vi "Lockin_Amplifier_save_diag.vi"(0 "Reference signal (dialog if empty)":path=path "D:/#Meresek/Malaria/Malaria_measurement_program/Labview/Lock_in_Amplifier/tesztsor/timetrace_46.txt", 1 "averaging time":dbl=1.0 format="%0.2p", 2 "tolerance (Deviation)":dbl=3.0, 5 "Sample Number":i32=100000, 7 "dt":dbl=0.0002, 9 "Window (s)":dbl=3.0, 11 "Resolution":dbl=1e-05, 12 "Error In":errorcluster) -> (3 "LD_RMS":dbl, 4 "Lock-in R":cluster{dbl[], "Result":dbl[]}(graph), 6 "Lock-in Theta":cluster{dbl[], "Result":dbl[]}(graph), 8 "LD mean (V)":dbl format="%0.6f", 10 "LD deviation (V)":dbl format="%0.6f", 13 "dLD_RMS":dbl, 14 "Error Out":errorcluster, 15 "Integral":cluster{dbl[], dbl[]}[](graph))   [LabVIEW 2011]
uses:
  <vilib>/Utility/file.llb/Read From Spreadsheet File (DBL).vi
  <vilib>/Utility/file.llb/Write To Spreadsheet File (DBL).vi
  <vilib>/gmath/NI_Gmath.lvlib
  <vilib>/Analysis/NI_AALBase.lvlib
panel:
  in  "Tab Control":T1(tab)
  out "Reference signal / PLL Signal":cluster{"all rows":dbl[], "all rows":dbl[]}[](graph)
  out "Reference Spectrum":cluster{"f0":dbl, "df":dbl, "magnitude":dbl[]}(graph)
  out "Synthetized Spectrum":cluster{"f0":dbl, "df":dbl, "magnitude":dbl[]}(graph)
  in  "t0_ref":dbl
  in  "t0_LD":dbl=0.0001
  in  "Sampling Freq":dbl=5000.0
  in  "Cutoff Frequency":dbl=500.0
  out "Averaging window":dbl
  in  "SAVE":path=path "D:/#Meresek/Malaria/Malaria_measurement_program/Labview/Lock_in_Amplifier/tesztsor/timetrace_46.txt"
  out "LD Spectrum":cluster{"f0":dbl, "df":dbl, "magnitude":dbl[]}(graph)
  out "LD Signal":cluster{"all rows":dbl[], "all rows":dbl[]}[](graph)
  out "Signal Spectrum":cluster{"f0":dbl, "df":dbl, "magnitude":dbl[]}[](graph)
  out "Time Domain Signal":cluster{"xi used":dbl[], "yi":dbl[]}[](graph)
  out "Tolerance Level":dbl
  out "average":dbl
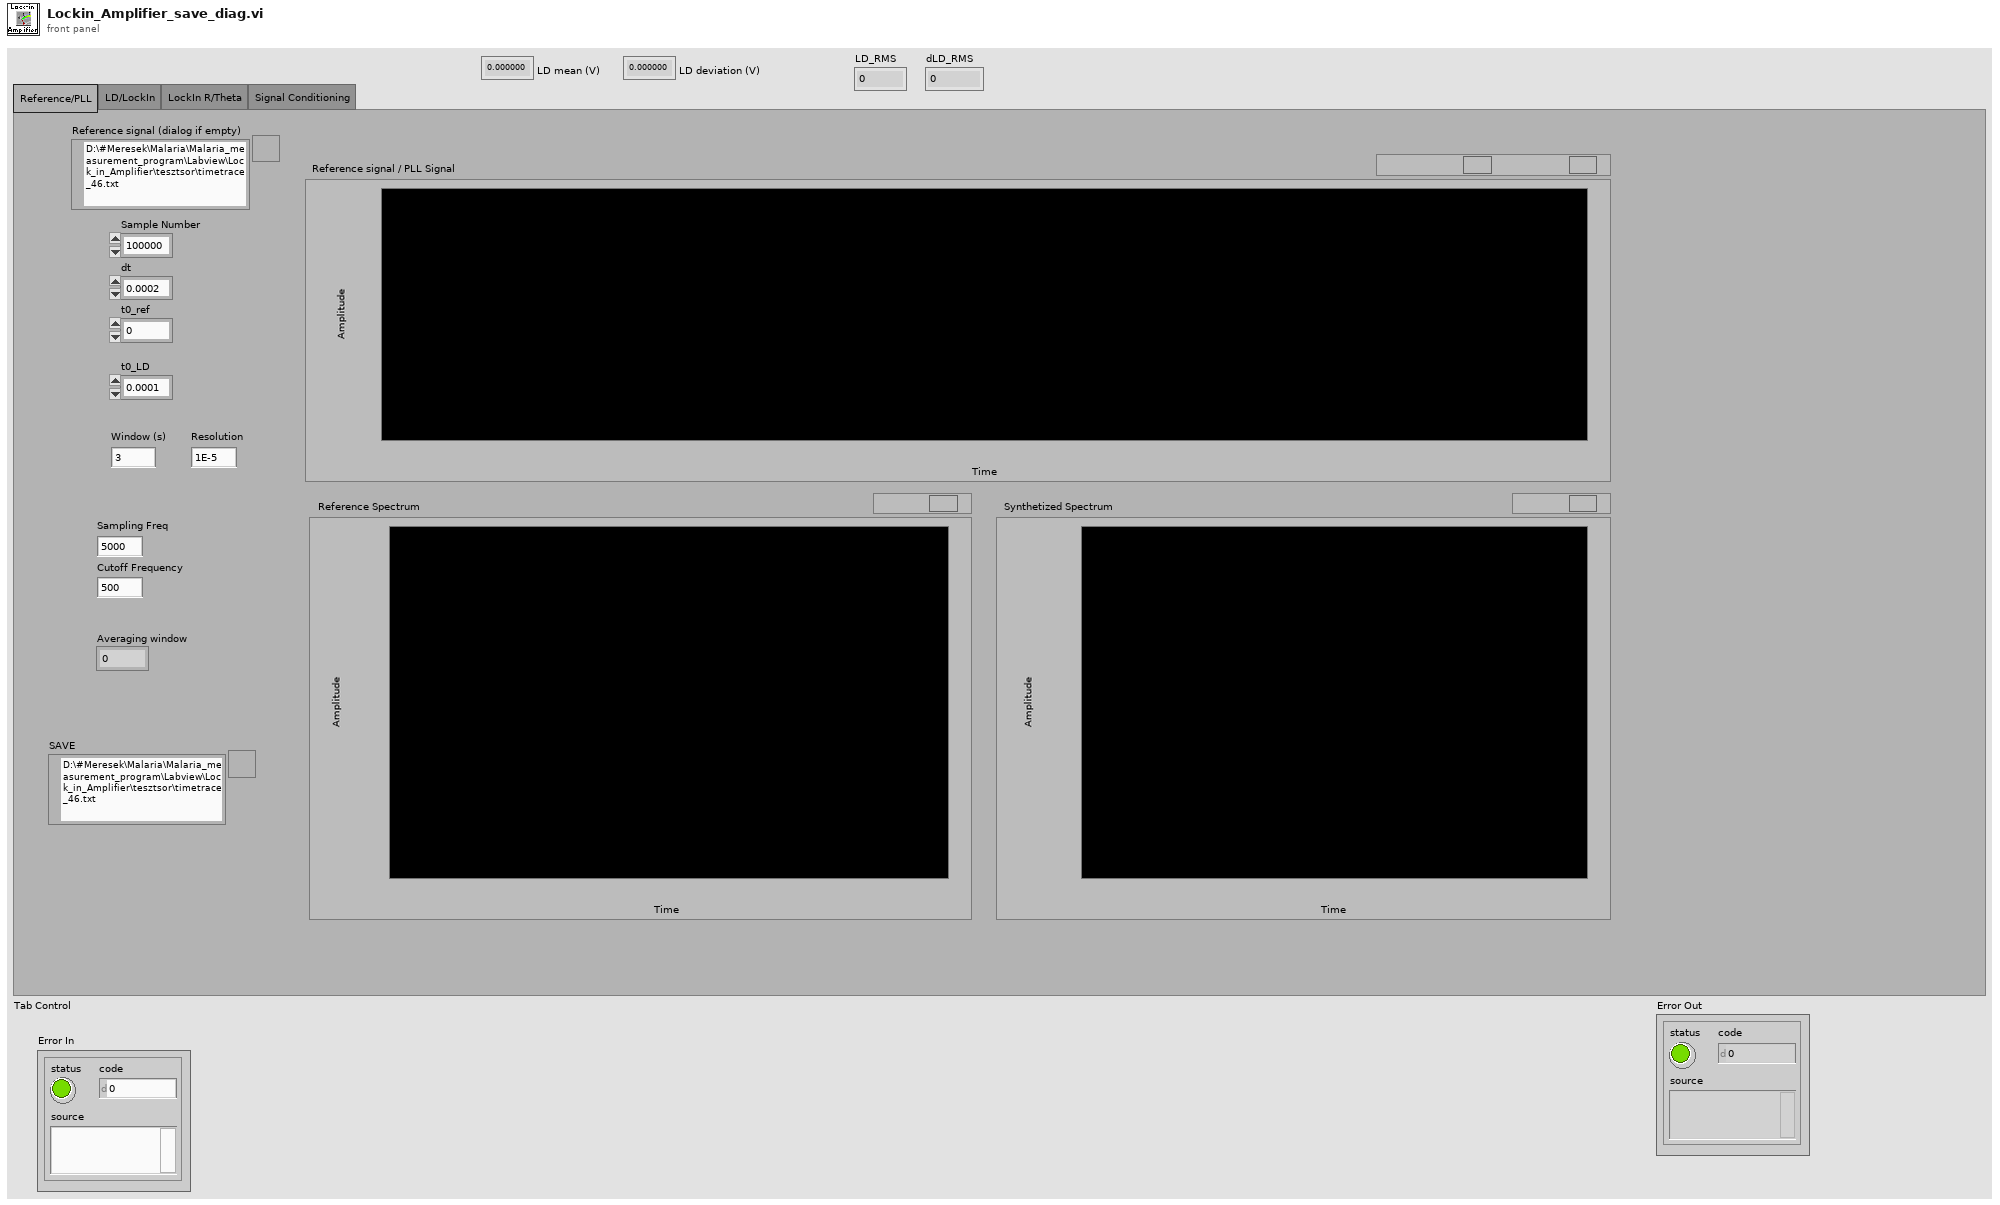
[diagram p1: front panel]
types:
  T1 = enum32{"Reference/PLL", "LD/LockIn", "LockIn R/Theta", "Signal Conditioning"}
  T2 = enum16{"open", "replace", "create", "open or create", "replace or create", "replace or create with confirmation"}
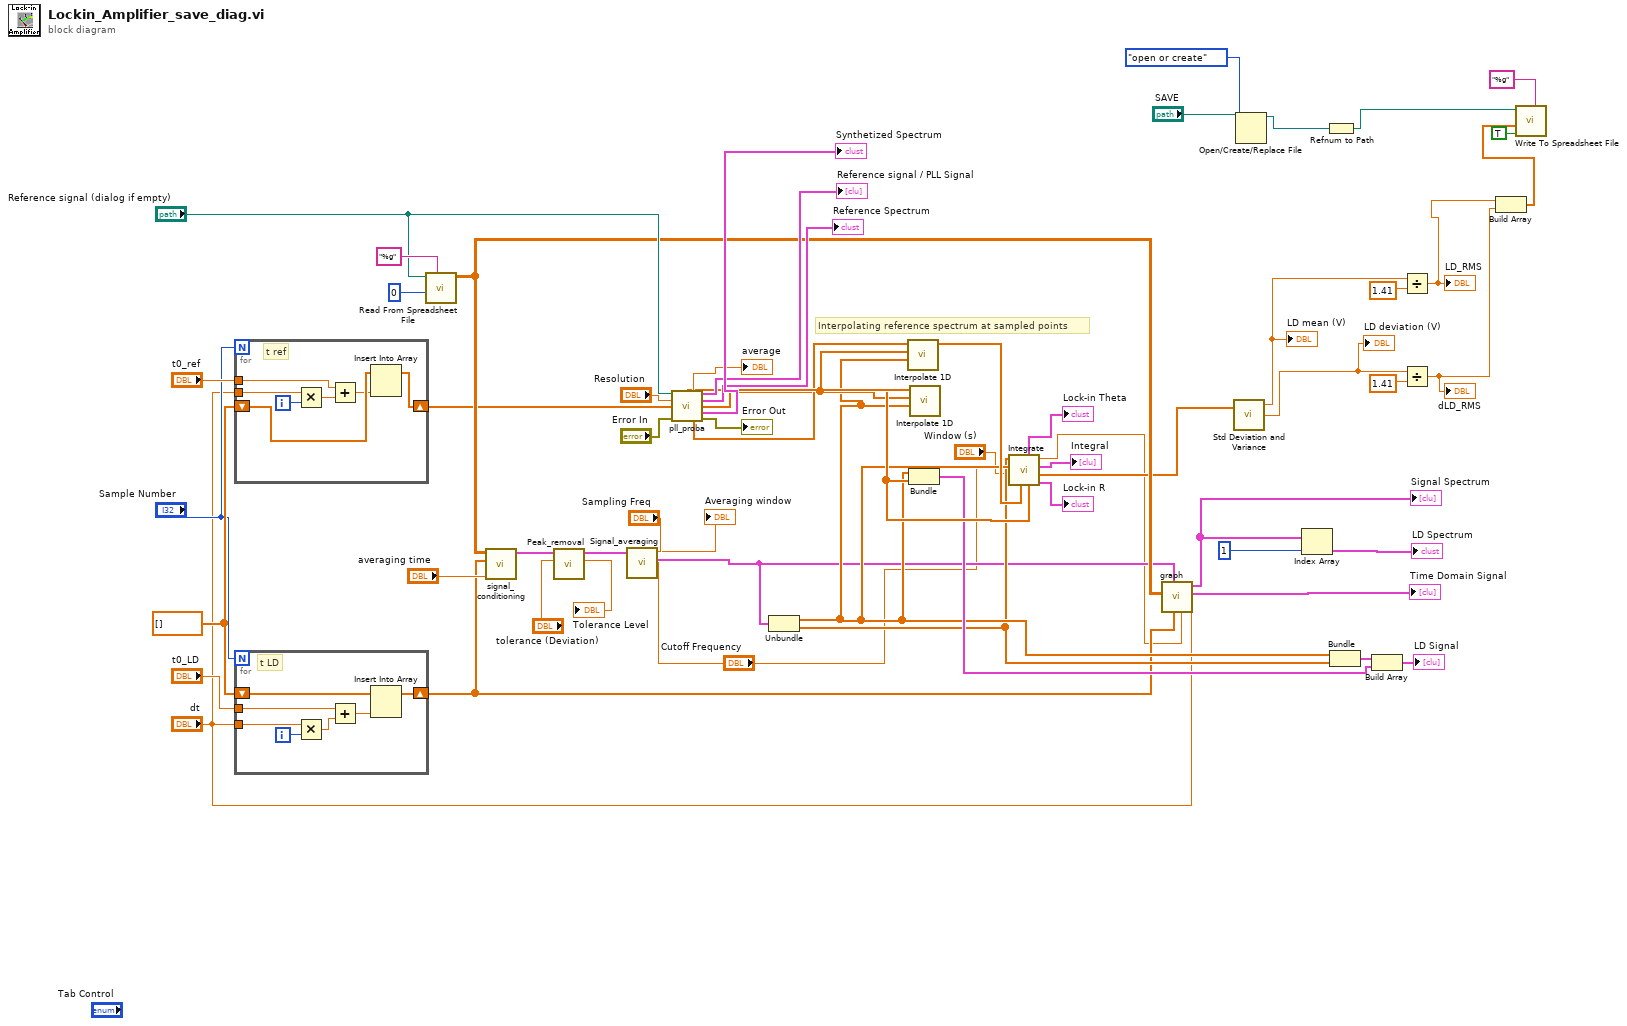
[diagram p0: block diagram]
diagram:
  w31 = dbl[] []
  # "Interpolating reference spectrum at sampled points"
  n1 = for {
    N: "Sample Number" -> [_]
    shift-right: [w66] -> w32
    shift-left: w31 -> [w65]
    tunnel: "dt" -> [w64]
    tunnel: "t0_ref" -> [w63]
    i -> [w67]
    # "t ref"
    n2 = Multiply(x=w64, y=w67) -> (x*y=w62:dbl)
    n3 = Add(x=w63, y=w62) -> (x+y=w61:dbl)
    n4 = Insert Into Array(array=w65, new element=w61) -> (w66:dbl[])  [unwired: 1 in]
  }
  n5 = for {
    N: "Sample Number" -> [_]
    shift-right: [w73] -> w28
    shift-left: w31 -> [w72]
    tunnel: "dt" -> [w71]
    tunnel: "t0_LD" -> [w70]
    i -> [w74]
    # "t LD"
    n6 = Multiply(x=w71, y=w74) -> (x*y=w69:dbl)
    n7 = Add(x=w70, y=w69) -> (x+y=w68:dbl)
    n8 = Insert Into Array(array=w72, new element=w68) -> (w73:dbl[])  [unwired: 1 in]
  }
  n9 = call-poly <vilib>:"Read From Spreadsheet File.vi"("format (%.3f)"="%g" ("format (%.6f)"), "start of read offset (chars.:0)"=0, "file path (dialog if empty)"="Reference signal (dialog if empty)") -> ("all rows"=w40:dbl[][])  [unwired: 4 in, 4 out]
  n10 = call "signal_conditioning.vi"("averaging time"="averaging time", "t_LD"=w28, "all rows"=w40) -> ("Offset removed"=w34:cluster{"xi used":dbl[], "yi":dbl[]})  [unwired: 7 in, 1 out]
  n11 = call "Peak_removal.vi"("tolerance (Deviation)"="tolerance (Deviation)", "Offset removed"=w34) -> ("Tolerance Level"=→"Tolerance Level":dbl, "XY Graph"=w21:cluster{"xi used":dbl[], "yi":dbl[]})  [unwired: 8 in]
  n12 = call "Signal_averaging.vi"("Pike removed"=w21, "Cutoff Frequency"="Cutoff Frequency", "Sampling Freq"="Sampling Freq") -> ("Averaged"=w20:cluster{"xi used":dbl[], "yi":dbl[]}, "Averaging window"=→"Averaging window":dbl)  [unwired: 7 in]
  n13 = call "pll_proba.vi"("Reference signal (dialog if empty)"="Reference signal (dialog if empty)", "Resolution"="Resolution", "t_ref"=w32, "Error In"="Error In") -> ("average"=→"average":dbl, "XY Graph"=→"Reference signal / PLL Signal":cluster{"all rows":dbl[], "all rows":dbl[]}[], "Waveform Graph"=→"Reference Spectrum":cluster{"f0":dbl, "df":dbl, "magnitude":dbl[]}, "time"=w43:dbl[], "Waveform Graph 2"=→"Synthetized Spectrum":cluster{"f0":dbl, "df":dbl, "magnitude":dbl[]}, "PLL_sine"=w47:dbl[], "PLL_cosine"=w44:dbl[], "Error Out"=→"Error Out":errorcluster)  [unwired: 4 in]
  n14 = Unbundle(w20) -> ("xi used"=w38:dbl[], "yi"=w37:dbl[])
  n15 = call <vilib>:"Interpolate 1D.vi"("xi"=w38, "X"=w43, "Y"=w44) -> ("yi"=w42:dbl[])  [unwired: 6 in, 2 out]
  n16 = call <vilib>:"Interpolate 1D.vi"("xi"=w38, "X"=w43, "Y"=w47) -> ("yi"=w46:dbl[])  [unwired: 6 in, 2 out]
  n17 = Bundle("xi used"=w38, "yi"=w46) -> (w45:cluster{"xi used":dbl[], "yi":dbl[]})  [unwired: 1 in]
  n18 = call "Integrate.vi"("yi 3"=w46, "yi 2"=w42, "Processed LD time values"=w38, "Window (s)"="Window (s)", "Cutoff Frequency"="Cutoff Frequency", "Processed LD values"=w37) -> ("LockIn R"=→"Lock-in R":cluster{dbl[], "Result":dbl[]}, "LockIn R array"=w26:dbl[], "Lock in X,Y,R time"=→"Integral":cluster{dbl[], "Result":dbl[]}[], "Numeric"=w15:dbl, "Lockin Theta"=→"Lock-in Theta":cluster{dbl[], "Result":dbl[]})  [unwired: 1 in]
  n19 = call "graph.vi"(4:"dt"=w15, "Array in"=w28, "Averaged"=w20, "LD Timetrace in"=w40, 11:"dt"="dt") -> ("Time Domain Signal"=→"Time Domain Signal":cluster{"xi used":dbl[], "yi":dbl[]}[], "Spectra"=w12:cluster{"f0":dbl, "df":dbl, "magnitude":dbl[]}[])  [unwired: 5 in]
  "Signal Spectrum" <- w12
  n20 = call <vilib>:"Std Deviation and Variance.vi"("X"=w26) -> ("mean"=w25:dbl, "standard deviation"=w22:dbl)  [unwired: 1 in, 1 out]
  "LD mean (V)" <- w25
  "LD deviation (V)" <- w22
  n21 = Open/Create/Replace File(file path (use dialog)="SAVE", operation (0:open)=T2."open or create") -> (refnum out=w5:refnum<file>)  [unwired: 4 in, 2 out]
  n22 = Index Array(array=w12, index=1) -> (element=→"LD Spectrum":cluster{"f0":dbl, "df":dbl, "magnitude":dbl[]})
  n23 = Refnum to Path(1:w5) -> (0:w4:path)
  n24 = Bundle("xi used"=w38, "yi"=w37) -> (w48:cluster{"xi used":dbl[], "yi":dbl[]})  [unwired: 1 in]
  n25 = Build Array(w48, w45) -> (→"LD Signal":cluster{"xi used":dbl[], "yi":dbl[]}[])
  n26 = Divide(x=w25, y=1.41) -> (x/y=w7:dbl)
  "LD_RMS" <- w7
  n27 = Divide(x=w22, y=1.41) -> (x/y=w6:dbl)
  "dLD_RMS" <- w6
  n28 = Build Array(w7, w6) -> (w3:dbl[])
  n29 = call-poly <vilib>:"Write To Spreadsheet File.vi"("format (%.3f)"="%g", "append to file? (new file:F)"=TRUE, "1D data"=w3, "file path (dialog if empty)"=w4) -> ()  [unwired: 4 in, 1 out]
